vi "Daxsonics.vi"() -> ()   [LabVIEW 2022 SP3]
doc: "This application VI allows the user to set the desired parameters in the \n5800 / 5900 P / R. just select thevalues that you want to set the instrument to from the 5800 / 5900 user interface and click on the send to 5800 button."
uses:
  ScanningControl/Pulsers/PulserGlobals.vi
panel:
  in  "Lock/Unlock":bool
  in  "ExitSendCmd":bool
  in  "Freq (MHz)":u16(ring)=1 items=["4", "6", "8", "10", "12", "15", "17", "20", "25", "30", "35", "40", "45", "50"]
  in  "CLK":u16(ring) items=["EXT", "INT"]
  in  "Period (us)":u16(ring) items=["1000"]
  in  "Amp (V)":u16(ring) items=["0", "15", "20", "25", "30", "35", "40", "45", "50", "55", "60", "65", "70", "75", "80", "85", "90", "95", "100"]
  in  "Gain (dB)":u16(ring) items=["0", "3", "6", "9", "12", "15", "18", "21", "24", "27", "30", "33", "36", "39", "42", "45"]
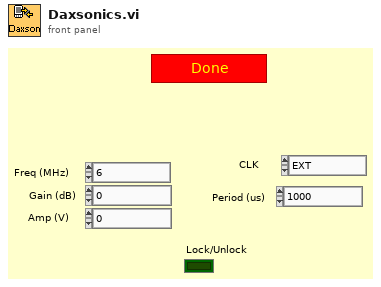
[diagram p1: front panel]
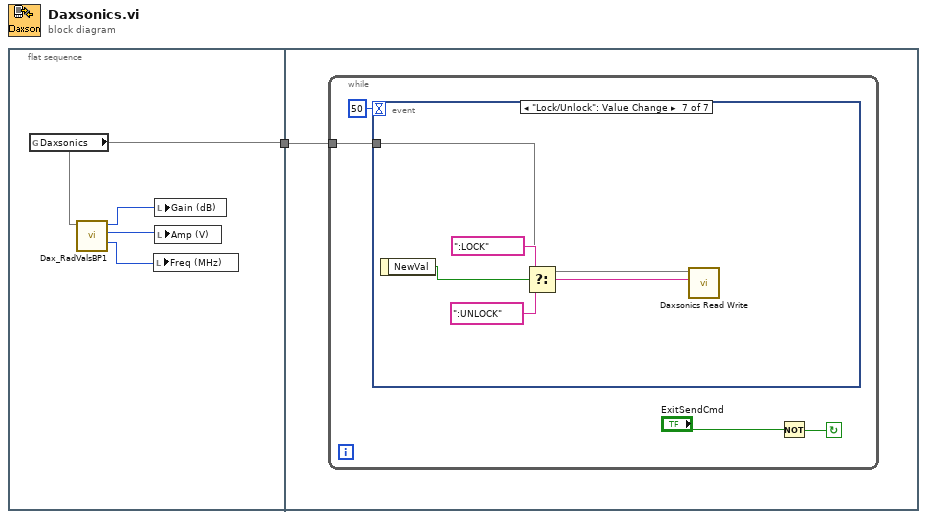
[diagram p0: block diagram]
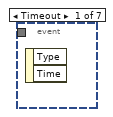
[diagram p2: hidden frame]
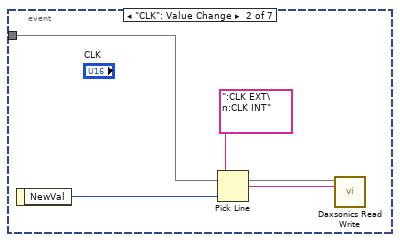
[diagram p3: hidden frame]
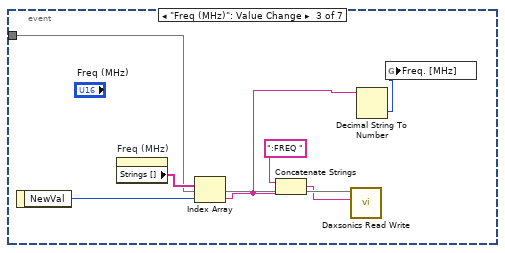
[diagram p4: hidden frame]
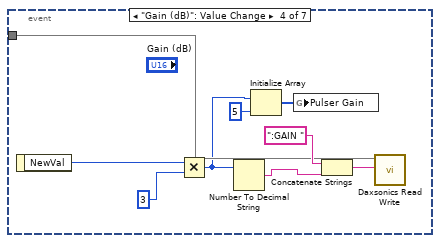
[diagram p5: hidden frame]
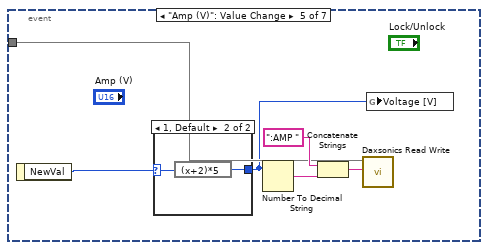
[diagram p6: hidden frame]
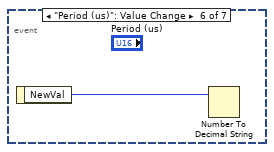
[diagram p8: hidden frame]
diagram:
  n1 = flat-sequence {
    tunnel: [w2] -> w1
    tunnel: w1 -> [w6]
    frame #0 {
      n2 = global read "PulserGlobals.vi" "Daxsonics"() -> (w2)
      n3 = call "Dax_RadValsBP1.vi"("Daxsonics"=w2) -> ("Freq (MHz)"=w3:u16, "Amp (V)"=w5:u16, "Gain (dB)"=w4:u16)  [unwired: 7 in, 1 out]
      n4 = local write "Freq (MHz)"(w3) -> ()
      n5 = local write "Gain (dB)"(w4) -> ()
      n6 = local write "Amp (V)"(w5) -> ()
    }
    frame #1 {
      n7 = while {
        tunnel: w6 -> [w7]
        stop <- w10 continue-if-true
        n8 = event shown="[6] \"Lock/Unlock\": Value Change" {
          selector: _ -> [_ _ _ _ _ _ _]
          dyn-events: _ -> [_ _ _ _ _ _ _]
          timeout: 50 -> [_ _ _ _ _ _ _]
          tunnel: w7 -> [_ w11 w18 w25 w32 _ w41]
          event Timeout {
            n9 = event-data() -> ()  [unwired: 3 out]
          }
          event "CLK": Value Change {
            n10 = event-data() -> ("NewVal"=w12:u16)  [unwired: 1 out]
            n11 = Pick Line(multi-line string=":CLK EXT\n:CLK INT", line index=w12) -> (output string=w13:string)  [unwired: 1 in]
            n12 = call "Daxsonics Read Write.vi"("write buffer"=w13, "VISA resource name"=w11) -> ()  [unwired: 7 in, 3 out]
          }
          event "Freq (MHz)": Value Change {
            n13 = event-data() -> ("NewVal"=w20:u16)  [unwired: 1 out]
            n14 = property on="Freq (MHz)" class="Ring (strict)"() -> ("Strings []"=w21:string[])  [unwired: 2 in, 2 out]
            n15 = Index Array(array=w21, index=w20) -> (element=w16:string)
            n16 = Concatenate Strings(":FREQ " ("string"), w16) -> (w17:string)
            n17 = call "Daxsonics Read Write.vi"("write buffer"=w17, "VISA resource name"=w18) -> ()  [unwired: 7 in, 3 out]
            n18 = Decimal String To Number(string=w16) -> (number=w15:i32)  [unwired: 2 in, 1 out]
            n19 = global write "PulserGlobals.vi" "Freq. [MHz]"(w15) -> ()
          }
          event "Gain (dB)": Value Change {
            n20 = event-data() -> ("NewVal"=w29:u16)  [unwired: 1 out]
            n21 = Multiply(x=w29, y=3) -> (x*y=w23:i32)
            n22 = Number To Decimal String(number=w23) -> (decimal integer string=w28:string)  [unwired: 1 in]
            n23 = Initialize Array(w23, 5 ("index")) -> (w22:i32[])
            n24 = global write "PulserGlobals.vi" "Pulser Gain"(w22) -> ()
            n25 = Concatenate Strings(":GAIN " ("string"), w28) -> (w27:string)
            n26 = call "Daxsonics Read Write.vi"("write buffer"=w27, "VISA resource name"=w25) -> ()  [unwired: 7 in, 3 out]
          }
          event "Amp (V)": Value Change {
            n27 = event-data() -> ("NewVal"=w36:u16)  [unwired: 1 out]
            n28 = case shown="1, Default" w36 {
              selector: w36 -> [w37 w39]
              tunnel: [w37 w38] -> w31
              frame 0 {
              }
              frame 1, Default {
                n29 = expression code="(x+2)*5"(w39) -> (w38:u16)
              }
            }
            n30 = Number To Decimal String(number=w31) -> (decimal integer string=w35:string)  [unwired: 1 in]
            n31 = Concatenate Strings(":AMP " ("string"), w35) -> (w34:string)
            n32 = call "Daxsonics Read Write.vi"("write buffer"=w34, "VISA resource name"=w32) -> ()  [unwired: 7 in, 3 out]
            n33 = global write "PulserGlobals.vi" "Voltage [V]"(w31) -> ()
          }
          event "Period (us)": Value Change {
            n34 = event-data() -> ("NewVal"=w40:u16)  [unwired: 1 out]
            n35 = Number To Decimal String(number=w40) -> ()  [unwired: 1 in, 1 out]
          }
          event "Lock/Unlock": Value Change {
            n36 = event-data() -> ("NewVal"=w45:bool)  [unwired: 1 out]
            n37 = Select(t=":LOCK", s=w45, f=":UNLOCK") -> (s? t:f=w42:string)
            n38 = call "Daxsonics Read Write.vi"("write buffer"=w42, "VISA resource name"=w41) -> ()  [unwired: 7 in, 3 out]
          }
        }
        n39 = Not(x="ExitSendCmd") -> (.not. x?=w10:bool)
      }
    }
  }
